vi "3_3_(1).vi"() -> ()   [LabVIEW 2012]
uses:
  Control 1.ctl
panel:
  in  "Зчитати дані":bool
  out "Таблиця 1 - Вхідні дані":string[][](table)
  out "Таблиця 2 - Сортування":string[][](table)
  in  "4":bool
  in  "3":bool
  in  "2":bool
  in  "1":bool
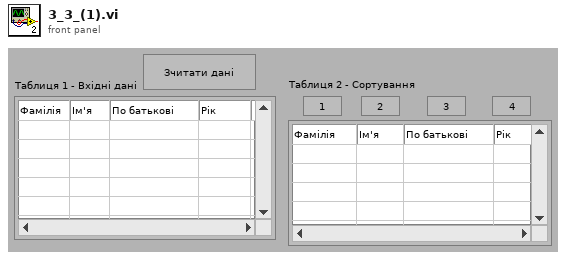
[diagram p1: front panel]
types:
  T1 = typedef "Control 1.ctl" = enum16{"Серверу", "Клієнту", "Зчитати", "Стоп", "1", "2", "3", "4"}
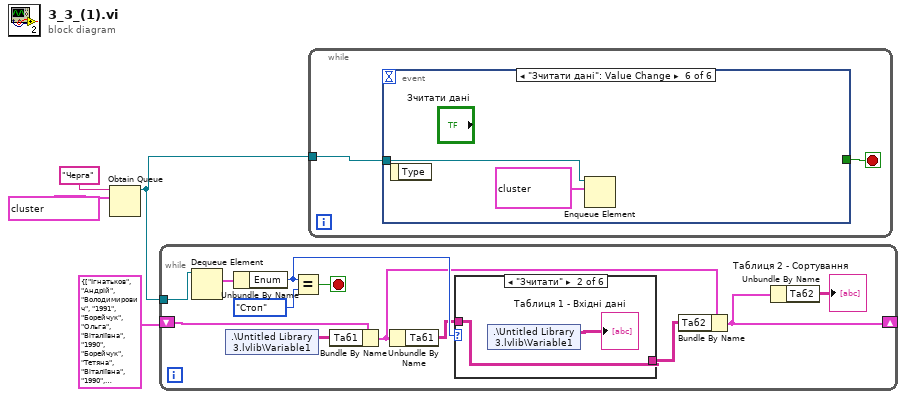
[diagram p0: block diagram]
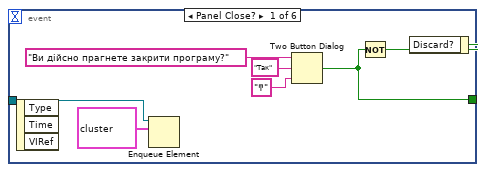
[diagram p2: hidden frame]
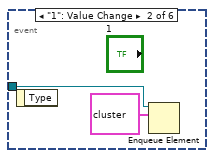
[diagram p3: hidden frame]
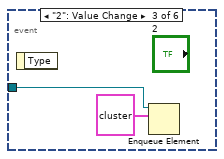
[diagram p4: hidden frame]
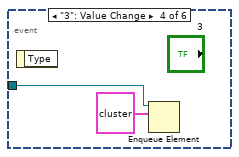
[diagram p5: hidden frame]
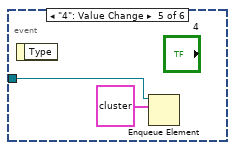
[diagram p6: hidden frame]
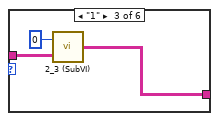
[diagram p8: hidden frame]
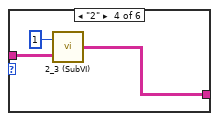
[diagram p9: hidden frame]
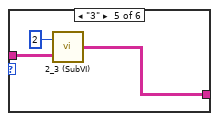
[diagram p10: hidden frame]
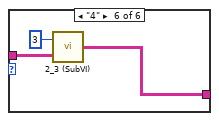
[diagram p11: hidden frame]
diagram:
  n1 = Obtain Queue(name (unnamed)="Черга", element data type=cluster{"variant":variant, "Enum":T1} {"variant"=variant, "Enum"=enum."Стоп"}) -> (queue out=w2:refnum<queue>)  [unwired: 3 in, 2 out]
  n2 = while {
    tunnel: w2 -> [w16]
    shift-right: [w10] -> _
    shift-left: cluster{"Таб1":string[][], "Таб2":string[][]} {"Таб1"=[["Ігнатьков", "Андрій", "Володимирович", "1991"], ["Борейчук", "Ольга", "Віталіївна", "1990"], ["Борейчук", "Тетяна", "Віталіївна", "1990"], ["Котлубаєв", "Максим", "Євгенович", "1991"], ["Котлуьаєв", "Віталій", "Євгенович", "1989"]], "Таб2"=[["Ігнатьков", "Андрій", "Володимирович", "1991"], ["Борейчук", "Ольга", "Віталіївна", "1990"], ["Борейчук", "Тетяна", "Віталіївна", "1990"], ["Котлубаєв", "Максим", "Євгенович", "1991"], ["Котлуьаєв", "Віталій", "Євгенович", "1989"]]} -> [w7]
    stop <- w13 stop-if-true
    n3 = Dequeue Element(queue=w16) -> (element=w15:cluster{"variant":variant, "Enum":T1})  [unwired: 2 in, 3 out]
    n4 = shared-variable ".\\Untitled Library 3.lvlib\\Variable1"() -> (w5:string[][])  [unwired: 1 in, 1 out]
    n5 = Unbundle By Name(w15) -> ("Enum"=w12:T1)
    n6 = Equal?(x=w12, y=Control_1."Стоп" ("Enum")) -> (x = y?=w13:bool)
    n7 = Bundle By Name(cluster=w7, "Таб1"=w5) -> (w6:cluster{"Таб1":string[][], "Таб2":string[][]})
    n8 = Unbundle By Name(w6) -> ("Таб1"=w11:string[][])
    n9 = case shown="\"Зчитати\"" w12 {
      tunnel: w11 -> [w17 w19 w22 w23 w26 w30]
      tunnel: [w17 w19 w20 w25 w28 w29] -> w8
      frame "Стоп", Default {
      }
      frame "Зчитати" {
        n10 = shared-variable ".\\Untitled Library 3.lvlib\\Variable1"() -> (→"Таблиця 1 - Вхідні дані":string[][])  [unwired: 1 in, 1 out]
      }
      frame "1" {
        n11 = call "2_3 (SubVI).vi"("Таблиця 1 - Вхідні дані"=w22, "Сортувати стовпчик"=0) -> ("Таблиця 2 - Результат"=w20:string[][])
      }
      frame "2" {
        n12 = call "2_3 (SubVI).vi"("Таблиця 1 - Вхідні дані"=w23, "Сортувати стовпчик"=1) -> ("Таблиця 2 - Результат"=w25:string[][])
      }
      frame "3" {
        n13 = call "2_3 (SubVI).vi"("Таблиця 1 - Вхідні дані"=w26, "Сортувати стовпчик"=2) -> ("Таблиця 2 - Результат"=w28:string[][])
      }
      frame "4" {
        n14 = call "2_3 (SubVI).vi"("Таблиця 1 - Вхідні дані"=w30, "Сортувати стовпчик"=3) -> ("Таблиця 2 - Результат"=w29:string[][])
      }
    }
    n15 = Bundle By Name(cluster=w6, "Таб2"=w8) -> (w10:cluster{"Таб1":string[][], "Таб2":string[][]})
    n16 = Unbundle By Name(w10) -> ("Таб2"=→"Таблиця 2 - Сортування":string[][])
  }
  n17 = while {
    tunnel: w2 -> [w32]
    stop <- w33 stop-if-true
    n18 = event shown="[5] \"Зчитати дані\": Value Change" {
      selector: _ -> [_ _ _ _ _ _]
      dyn-events: _ -> [_ _ _ _ _ _]
      timeout: _ -> [_ _ _ _ _ _]
      tunnel: [w36 _ _ _ _ _] -> w33
      tunnel: w32 -> [w35 w41 w43 w45 w47 w49]
      event Panel Close? {
        n19 = event-data() -> ()  [unwired: 1 in, 3 out]
        n20 = Enqueue Element(queue=w35, element=cluster{"variant":variant, "Enum":T1} {"variant"=variant, "Enum"=enum."Стоп"}) -> ()  [unwired: 2 in, 3 out]
        n21 = Two Button Dialog(message="Ви дійсно прагнете закрити програму?", 1:"ͳ" ("F button name (\"Cancel\")"), 2:"Так" ("T button name (\"OK\")")) -> (T button?=w36:bool)
        n22 = Not(x=w36) -> (.not. x?=w37:bool)
        n23 = event-data("Discard?"=w37) -> ()  [unwired: 1 in, 1 out]
      }
      event "1": Value Change {
        n24 = event-data() -> ()  [unwired: 1 in, 1 out]
        n25 = Enqueue Element(queue=w41, element=cluster{"variant":variant, "Enum":T1} {"variant"=variant, "Enum"=enum."1"}) -> ()  [unwired: 2 in, 3 out]
      }
      event "2": Value Change {
        n26 = event-data() -> ()  [unwired: 1 in, 1 out]
        n27 = Enqueue Element(queue=w43, element=cluster{"variant":variant, "Enum":T1} {"variant"=variant, "Enum"=enum."2"}) -> ()  [unwired: 2 in, 3 out]
      }
      event "3": Value Change {
        n28 = event-data() -> ()  [unwired: 1 in, 1 out]
        n29 = Enqueue Element(queue=w45, element=cluster{"variant":variant, "Enum":T1} {"variant"=variant, "Enum"=enum."3"}) -> ()  [unwired: 2 in, 3 out]
      }
      event "4": Value Change {
        n30 = event-data() -> ()  [unwired: 1 in, 1 out]
        n31 = Enqueue Element(queue=w47, element=cluster{"variant":variant, "Enum":T1} {"variant"=variant, "Enum"=enum."4"}) -> ()  [unwired: 2 in, 3 out]
      }
      event "Зчитати дані": Value Change {
        n32 = event-data() -> ()  [unwired: 1 in, 1 out]
        n33 = Enqueue Element(queue=w49, element=cluster{"variant":variant, "Enum":T1} {"variant"=variant, "Enum"=enum."Зчитати"}) -> ()  [unwired: 2 in, 3 out]
      }
    }
  }
